vi "Actor Core.vi"(8 "error in":errorcluster, 11 "ServerUI in":refnum<class "ServerUI.lvclass">) -> (0 "error out":errorcluster, 3 "Actor out":refnum<class "Actor.lvclass">)   [LabVIEW 2018, in "ServerUI.lvlib" / "ServerUI.lvclass"]
doc: "(<B>Filename</B>: Actor Framework.lvlib:Actor.lvclass:Actor Core.vi)\n\nReceives messages to the actor, reacts to them, and initiates any error handling that may shut the actor down.\n\nDescendant classes may override this VI to append parallel tasks for the actor to complete while it handles messages. Overrides use the Call Parent Method node."
uses:
  ServerUI.lvclass
  C:/Program Files/National Instruments/LabVIEW 2018/vi.lib/ActorFramework/Actor/Actor.lvclass
  <vilib>/ActorFramework/Actor/Actor.lvclass
  <vilib>/ActorFramework/Actor/Actor.lvclass/Actor.ctl
  <vilib>/ActorFramework/Message Enqueuer/Message Enqueuer.lvclass/Message Enqueuer.ctl
  ServerUI.lvclass/ServerUI.ctl
  TCP_Client/TCP_Client Messages/Write Msg/Write Msg.lvclass/Write Msg.ctl
  <vilib>/ActorFramework/Message Enqueuer/Init from Existing Queue.vi
  <vilib>/ActorFramework/Message Enqueuer/Enqueue.vi
  TCP_Client/TCP_Client Messages/Write Msg/Write Msg.lvclass
  C:/Program Files/National Instruments/LabVIEW 2018/vi.lib/ActorFramework/Message/Message.lvclass
  <vilib>/ActorFramework/Stop Msg/Stop Msg.lvclass
  <vilib>/ActorFramework/Message Priority Queue/Priority Enqueue.vi
  <vilib>/ActorFramework/Message Enqueuer/Message Enqueuer.lvclass
  TCP_Server/TCP_Server/TCP_Server.lvclass
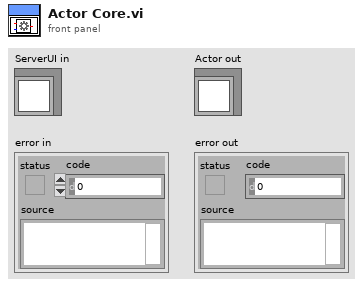
[diagram p1: front panel]
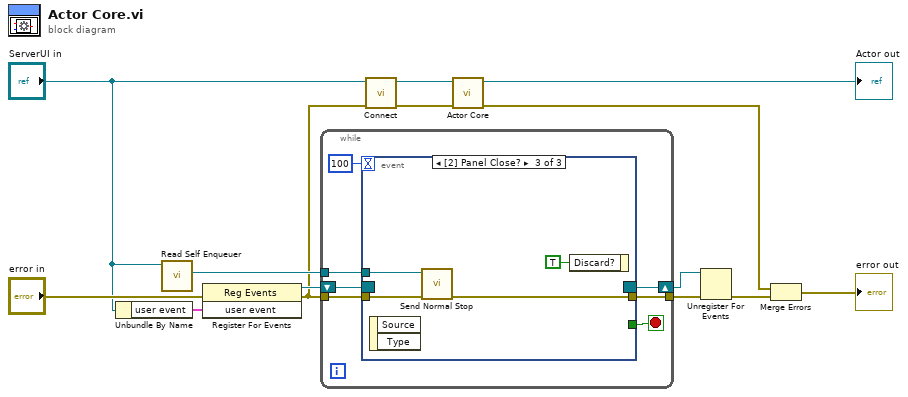
[diagram p0: block diagram]
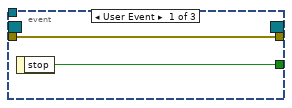
[diagram p2: hidden frame]
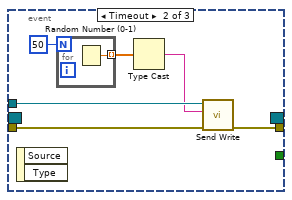
[diagram p3: hidden frame]
diagram:
  n1 = Unbundle By Name("ServerUI in") -> ("user event"=w12:cluster{"stop":refnum<user-event>})
  n2 = call <vilib>:"Read Self Enqueuer.vi"("Actor"="ServerUI in") -> ("Self Enqueuer"=w5:refnum<class "Message Enqueuer.lvclass">)  [unwired: 10 in]
  n3 = register-events(error in="error in", w12) -> (reference out=w11:refnum<event-registration>, error out=w1:errorcluster)  [unwired: 1 in]
  n4 = while {
    shift-right: [w18] -> w9
    shift-left: w11 -> [w21]
    tunnel: w1 -> [w20]
    tunnel: [w19] -> w10
    tunnel: w5 -> [w16]
    stop <- w17 stop-if-true
    n5 = event shown="[2] Panel Close?" {
      selector: w21 -> [_ _ _]
      dyn-events: [_ _ _] -> w18
      timeout: 100 -> [_ _ _]
      tunnel: w20 -> [w23 w29 w32]
      tunnel: [w23 w28 w31] -> w19
      tunnel: [w22 _ _] -> w17
      tunnel: w16 -> [_ w27 w33]
      event User Event {
        n6 = event-data() -> ("stop"=w22:bool)  [unwired: 1 in]
      }
      event Timeout {
        n7 = event-data() -> ()  [unwired: 1 in, 2 out]
        n8 = for {
          N: 50 ("# of Points") -> [_]
          tunnel: [w30] -> w25 mode=indexing
          n9 = Random Number (0-1)() -> (number: 0 to 1=w30:dbl)
        }
        n10 = Type Cast(x=w25) -> (*(type *) &x=w24:string)  [unwired: 1 out]
        n11 = call "Send Write.vi"("error in (no error)"=w29, "Message"=w24, "Message Enqueuer"=w27) -> ("error out"=w28:errorcluster)  [unwired: 7 in, 1 out]
      }
      event Panel Close? {
        n12 = event-data() -> ()  [unwired: 1 in, 2 out]
        n13 = call <vilib>:"Send Normal Stop.vi"("error in (no error)"=w32, "Message Enqueuer"=w33) -> ("error out"=w31:errorcluster)  [unwired: 9 in]
        n14 = event-data("Discard?"=TRUE) -> ()  [unwired: 1 in, 1 out]
      }
    }
  }
  n15 = call-dynamic "Connect.vi"("error in (no error)"=w1, "TCP_Server in"="ServerUI in") -> ("error out"=w3:errorcluster, "TCP_Server out"=w4:refnum<class "ServerUI.lvclass">)  [unwired: 8 in]
  n16 = call-parent "Actor Core.vi"("error in"=w3, "Actor in"=w4) -> ("error out"=w14:errorcluster, "Actor out"=→"Actor out":refnum<class "Actor.lvclass">)  [unwired: 8 in]
  n17 = Unregister For Events(event registration refnum=w9, error in=w10) -> (error out=w6:errorcluster)
  n18 = Merge Errors(w14, w6) -> (→"error out":errorcluster)
